vi "Process Malleable VI Hierarchy.vi"(8 "error in (no error)":errorcluster, 9 "Polymorphic Label":string, 10 "SubVI Ref In":refnum<vi>, 11 "Library Ref In":refnum<vi>) -> (0 "error out":errorcluster)   [LabVIEW 2020]
doc: "<b>This VI is recursive.</b>\n\nPerforms a depth first search for malleable VIs from the given subVI. When a vim with no malleable subVIs is found, it is converted to a polymorphic VI. As the function returns back up the tree, each malleable subVI reference is replaced with the matching polymorphic VI."
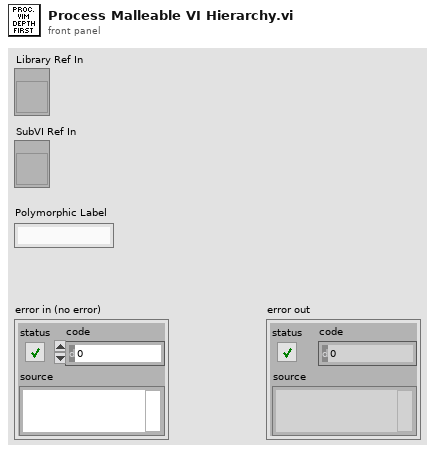
[diagram p1: front panel]
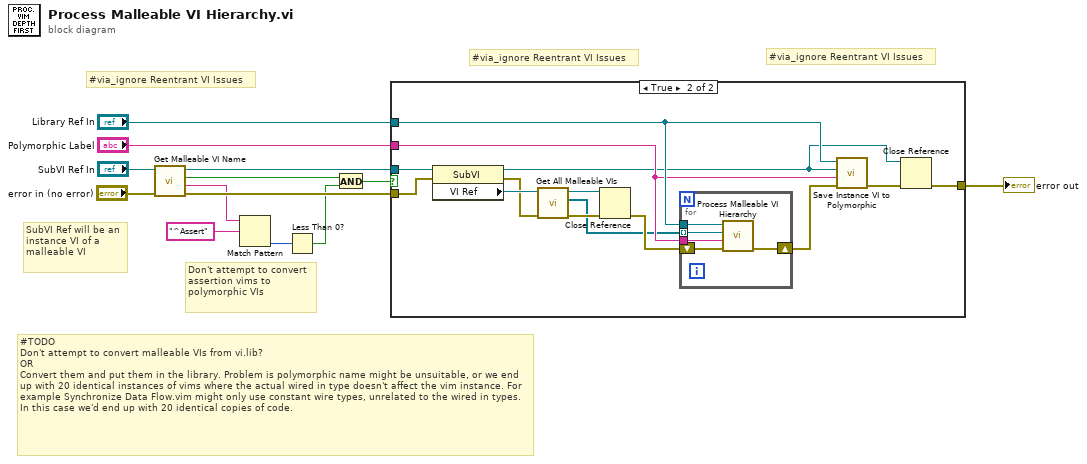
[diagram p0: block diagram]
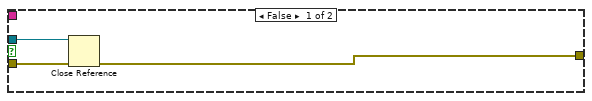
[diagram p2: hidden frame]
diagram:
  # "#via_ignore Reentrant VI Issues"
  # "#via_ignore Reentrant VI Issues"
  # "#via_ignore Reentrant VI Issues"
  # "#TODO\nDon't attempt to convert malleable VIs from vi.lib?\nOR\nConvert them and put them in the library. Problem is polymorphic name might be unsuitable, or we end up with 20 identical instances of vims where the actual wired in type doesn't affect the vim instance. For example Synchronize Data Flow.vim might only use constant wire types, unrelated to the wired in types. In this case we'd end up with 20 identical copies of code."
  # "Don't attempt to convert assertion vims to polymorphic VIs"
  # "SubVI Ref will be an instance VI of a malleable VI"
  n1 = call "Get Malleable VI Name.vi"("error in (no error)"="error in (no error)", "SubVI Ref In"="SubVI Ref In") -> ("error out"=w11:errorcluster, "Name without extension"=w7:string, "Is Malleable VI?"=w3:bool, "SubVI Ref Out"=w12:refnum<vi>)  [unwired: 5 in, 1 out]
  n2 = Match Pattern(string=w7, regular expression="^Assert") -> (offset past match=w5:i32)  [unwired: 1 in, 3 out]
  n3 = Less Than 0?(x=w5) -> (x < 0?=w4:bool)
  n4 = And(x=w3, y=w4) -> (x .and. y?=w1:bool)
  n5 = case shown="True" w1 {
    tunnel: w12 -> [w16 w23]
    tunnel: w11 -> [w14 w30]
    tunnel: "Polymorphic Label" -> [_ w19]
    tunnel: [w15 w21] -> w8
    tunnel: "Library Ref In" -> [_ w20]
    frame False {
      n6 = Close Reference(reference=w16, error in (no error)=w14) -> (error out=w15:errorcluster)
    }
    frame True {
      n7 = property on="Property Node" class="SubVI"(reference=w23, error in=w30) -> (reference out=w18:refnum<vi>, error out=w26:errorcluster, "VI Ref"=w28:refnum<vi>)
      n8 = call "Get All Malleable VIs.vi"("error in (no error)"=w26, "VI Ref In"=w28) -> ("error out"=w25:errorcluster, "Malleable VIs"=w17:refnum<vi>[], "VI Ref Out"=w27:refnum<vi>)  [unwired: 7 in]
      n9 = Close Reference(reference=w27, error in (no error)=w25) -> (error out=w24:errorcluster)
      n10 = for {
        tunnel: w17 -> [w32] mode=indexing
        tunnel: w19 -> [w33]
        shift-right: [w34] -> w29
        shift-left: w24 -> [w35]
        tunnel: w20 -> [w31]
        n11 = call "Process Malleable VI Hierarchy.vi"("error in (no error)"=w35, "Polymorphic Label"=w33, "SubVI Ref In"=w32, "Library Ref In"=w31) -> ("error out"=w34:errorcluster)  [unwired: 7 in]
      }
      n12 = call "Save Instance VI to Polymorphic.vi"("error in (no error)"=w29, "Polymorphic Label"=w19, "SubVI Ref In"=w18, "Library Ref In"=w20) -> ("error out"=w22:errorcluster)  [unwired: 7 in]
      n13 = Close Reference(reference=w18, error in (no error)=w22) -> (error out=w21:errorcluster)
    }
  }
  "error out" <- w8
